vi "calc running avg..vi"(8 "new val":dbl, 9 "reset?":bool, 11 "Averaging variables":T1) -> (0 "Average val":dbl, 3 "Averaging variables out":T1)   [LabVIEW 2019, in "Main.lvclass"]
doc: "Developed by Kevin Thompson\nkevin@thompsonengineering.net\n\nCopyright 2020\nThompson Engineering, LLC"
uses:
  Main.lvclass
  DataTypes/averaging variables.ctl
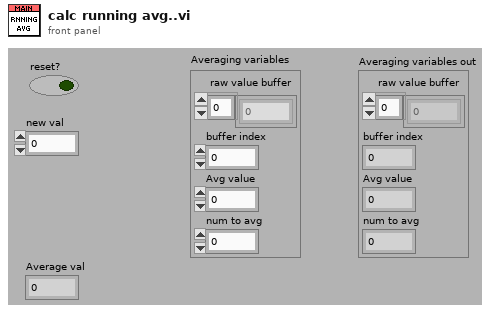
[diagram p1: front panel]
types:
  T1 = typedef "Main.lvclass/averaging variables.ctl" = cluster{"raw value buffer":dbl[], "buffer index":i32, "Avg value":dbl, "num to avg":i32}
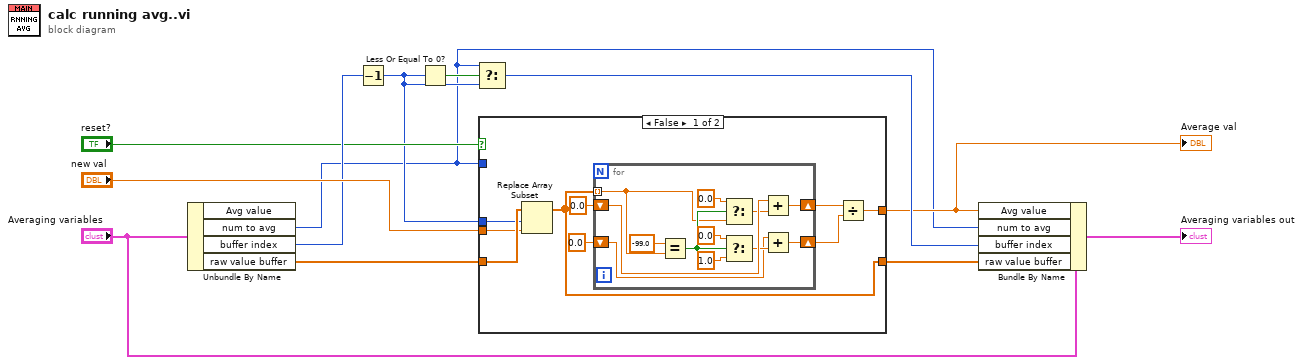
[diagram p0: block diagram]
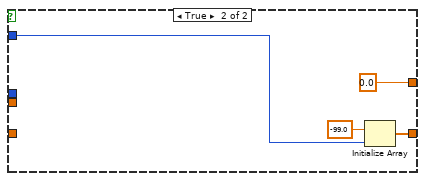
[diagram p2: hidden frame]
diagram:
  n1 = Unbundle By Name("Averaging variables") -> ("num to avg"=w1:i32, "buffer index"=w6:i32, "raw value buffer"=w8:dbl[])  [unwired: 1 out]
  n2 = Decrement(x=w6) -> (x-1=w3:i32)
  n3 = Less Or Equal To 0?(x=w3) -> (x <= 0?=w11:bool)
  n4 = Select(t=w1, s=w11, f=w3) -> (s? t:f=w10:i32)
  n5 = case shown="False" "reset?" {
    tunnel: w1 -> [_ w37]
    tunnel: [w17 0.0] -> w4
    tunnel: [w13 w34] -> w9
    tunnel: w8 -> [w16 _]
    tunnel: "new val" -> [w15 _]
    tunnel: w3 -> [w14 _]
    frame False {
      n6 = Replace Array Subset(array=w16, new element=w15, index=w14) -> (w13:dbl[])
      n7 = for {
        shift-right: [w29] -> w19
        shift-left: 0.0 ("new ESR calc") -> [w33]
        tunnel: w13 -> [w22] mode=indexing
        shift-right: [w25] -> w18
        shift-left: 0.0 -> [w26]
        n8 = Equal?(x=-99.0, y=w22) -> (x = y?=w28:bool)
        n9 = Select(t=0.0, s=w28, f=w22) -> (s? t:f=w31:dbl)
        n10 = Select(t=0.0, s=w28, f=1.0) -> (s? t:f=w27:dbl)
        n11 = Add(x=w33, y=w31) -> (x+y=w29:dbl)
        n12 = Add(x=w26, y=w27) -> (x+y=w25:dbl)
      }
      n13 = Divide(x=w19, y=w18) -> (x/y=w17:dbl)
    }
    frame True {
      n14 = Initialize Array(-99.0 ("element"), w37) -> (w34:dbl[])
    }
  }
  "Average val" <- w4
  n15 = Bundle By Name(cluster="Averaging variables", "Avg value"=w4, "num to avg"=w1, "buffer index"=w10, "raw value buffer"=w9) -> (→"Averaging variables out":T1)
